vi "Add PID.vi"(8 "error in (no error)":errorcluster, 11 "Node Ptr":u64 format="%.0x") -> (0 "error out":errorcluster)   [LabVIEW 2015, in "Diagnostics Addon System Explorer.lvlib"]
uses:
  Diagnostics Addon System Explorer.lvlib
  Shared/GUID Lookup.vi
  <vilib>/NI Veristand/Custom Device API/Custom Device API.lvlib
  Shared/Diagnostics Addon Shared.lvlib
  <vilib>/NI Veristand/Custom Device Tools/Custom Device Utility Library/Custom Device Utility Library.lvlib
panel:
  in  "Tag":string
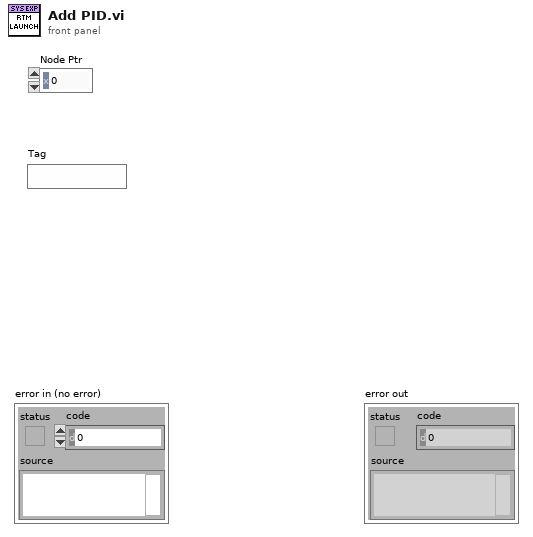
[diagram p1: front panel]
types:
  T1 = typedef "Custom Device API.lvlib/Custom Device Item Info.ctl" = cluster{"Name":string, "Is Channel":bool, "GUID":string, "Is Waveform":bool}
  T2 = typedef "Custom Device API.lvlib/Custom Device Item Ref.ctl" = u64
  T3 = typedef "Diagnostics Addon Shared.lvlib/DIDPID Parameters.ctl" = cluster{"Name":string, "Description":string, "ID":u16, "Signals":T4[]}
  T4 = typedef "Diagnostics Addon Shared.lvlib/DIDPID Signal Parameters.ctl" = cluster{"Start Bit":u8, "Length":u8, "Scaling Factor":dbl, "Scaling Offset":dbl, "Minimum":dbl, "Maximum":dbl, "Data Type":u32, "Byte Order":u32, "Default Value":dbl, "Name":string, "Units":string, "Description":string}
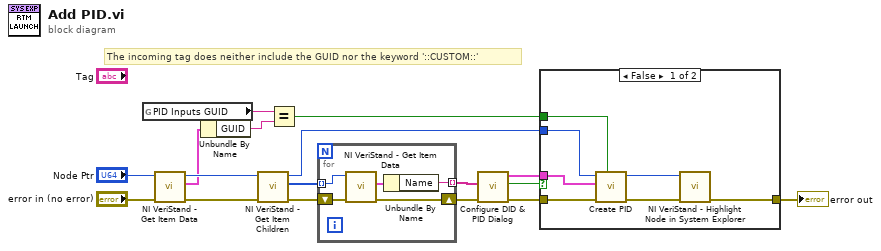
[diagram p0: block diagram]
diagram:
  # "The incoming tag does neither include the GUID nor the keyword '::CUSTOM::'"
  n1 = global read "GUID Lookup.vi" "PID Inputs GUID"() -> (w3:string)
  n2 = call <vilib>:"NI VeriStand - Get Item Data.vi"("error in (no error)"="error in (no error)", "Item Ref in"="Node Ptr") -> ("error out"=w7:errorcluster, "Item Info"=w4:T1, "Item Ref out"=w5:T2)  [unwired: 6 in, 1 out]
  n3 = Unbundle By Name(w4) -> ("GUID"=w2:string)
  n4 = call <vilib>:"NI VeriStand - Get Item Children.vi"("error in (no error)"=w7, "Item Ref in"=w5) -> ("error out"=w17:errorcluster, "Child Refs"=w10:T2[], "Item Ref out"=w9:T2)  [unwired: 6 in, 1 out]
  n5 = Equal?(x=w3, y=w2) -> (x = y?=w1:bool)
  n6 = for {
    tunnel: [w20] -> w16 mode=indexing
    shift-right: [w19] -> w15
    shift-left: w17 -> [w21]
    tunnel: w10 -> [w18] mode=indexing
    n7 = call <vilib>:"NI VeriStand - Get Item Data.vi"("error in (no error)"=w21, "Item Ref in"=w18) -> ("error out"=w19:errorcluster, "Item Info"=w22:T1)  [unwired: 8 out]
    n8 = Unbundle By Name(w22) -> ("Name"=w20:string)
  }
  n9 = call "Configure DID & PID Dialog.vi"("error in (no error)"=w15, "Existing PIDs"=w16) -> ("error out"=w13:errorcluster, "Cancel PID?"=w14:bool, "Parameters Out"=w12:T3)  [unwired: 7 in]
  n10 = case shown="False" w14 {
    tunnel: w13 -> [w29 w30]
    tunnel: w9 -> [w28 _]
    tunnel: w12 -> [w27 _]
    tunnel: [w23 w30] -> w11
    tunnel: w1 -> [w26 _]
    frame False {
      n11 = call "Create PID.vi"("Input?"=w26, "error in (no error)"=w29, "DIDPID"=w27, "Section Ptr"=w28) -> ("error out"=w24:errorcluster, "Parent Ref out"=w25:T2)  [unwired: 6 in]
      n12 = call <vilib>:"NI VeriStand - Highlight Node in System Explorer.vi"("error in (no error)"=w24, "Item Ref in"=w25) -> ("error out"=w23:errorcluster)  [unwired: 8 in, 1 out]
    }
    frame True {
    }
  }
  "error out" <- w11
